vi "syncAIandAOat1MHz_v3.vi"() -> ()   [LabVIEW 2015]
uses:
  <vilib>/DAQmx/write.llb/DAQmx Write (Digital 1D Wfm NChan NSamp).vi
  <vilib>/DAQmx/write.llb/DAQmx Write (Analog 1D Wfm NChan NSamp).vi
  <vilib>/DAQmx/read.llb/DAQmx Read (Analog 2D I16 NChan NSamp).vi
  <vilib>/Waveform/DWDTOps.llb/DWDT Analog to Digital.vi
  <vilib>/DAQmx/create/channels.llb/DAQmx Create Channel (AO-Voltage-Basic).vi
  <vilib>/DAQmx/create/channels.llb/DAQmx Create Channel (AI-Voltage-Basic).vi
  <vilib>/DAQmx/create/channels.llb/DAQmx Create Channel (DO-Digital Output).vi
  <vilib>/DAQmx/configure/timing.llb/DAQmx Timing (Sample Clock).vi
  <vilib>/Waveform/DWDTOps.llb/DWDT Uncompress Digital.vi
  <vilib>/DAQmx/miscellaneous.llb/DAQmx Fill In Error Info.vi
  <vilib>/DAQmx/configure/trigger.llb/DAQmx Start Trigger (Digital Edge).vi
  <resource>/objmgr/daqmx.rc
panel:
  in  "numcyc":dbl=9.0 format="%#_13g"
  in  "finite":bool
  in  "cont":bool
  in  "error in 3":errorcluster caption="error in"
  in  "index (page)":i32
  out "XY Graph":T1(graph)
  in  "V":dbl=2.0 format="%#_13g"
  in  "AOrate":dbl=400000.0 format="%#_13g"
  in  "stop":bool
  out "Intensity Graph":sgl[][](graph)
  in  "error in 2":errorcluster caption="error in"
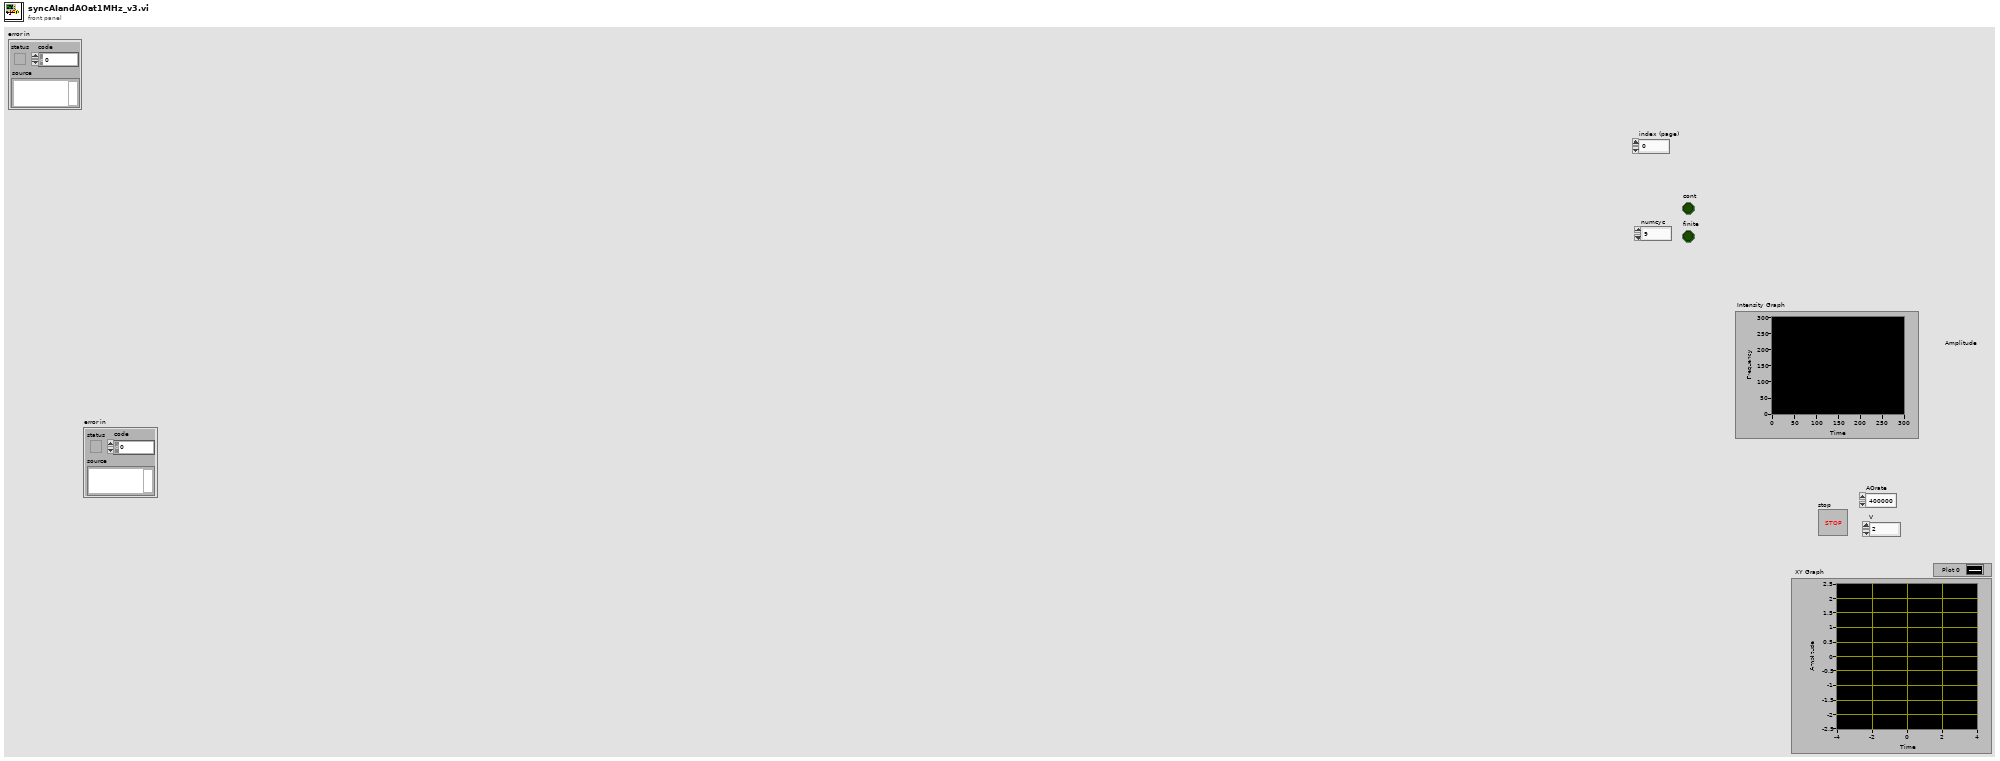
[diagram p1: front panel]
types:
  T1 = cluster{"X-WaveArray":dbl[], "Y-WaveArray":dbl[]}
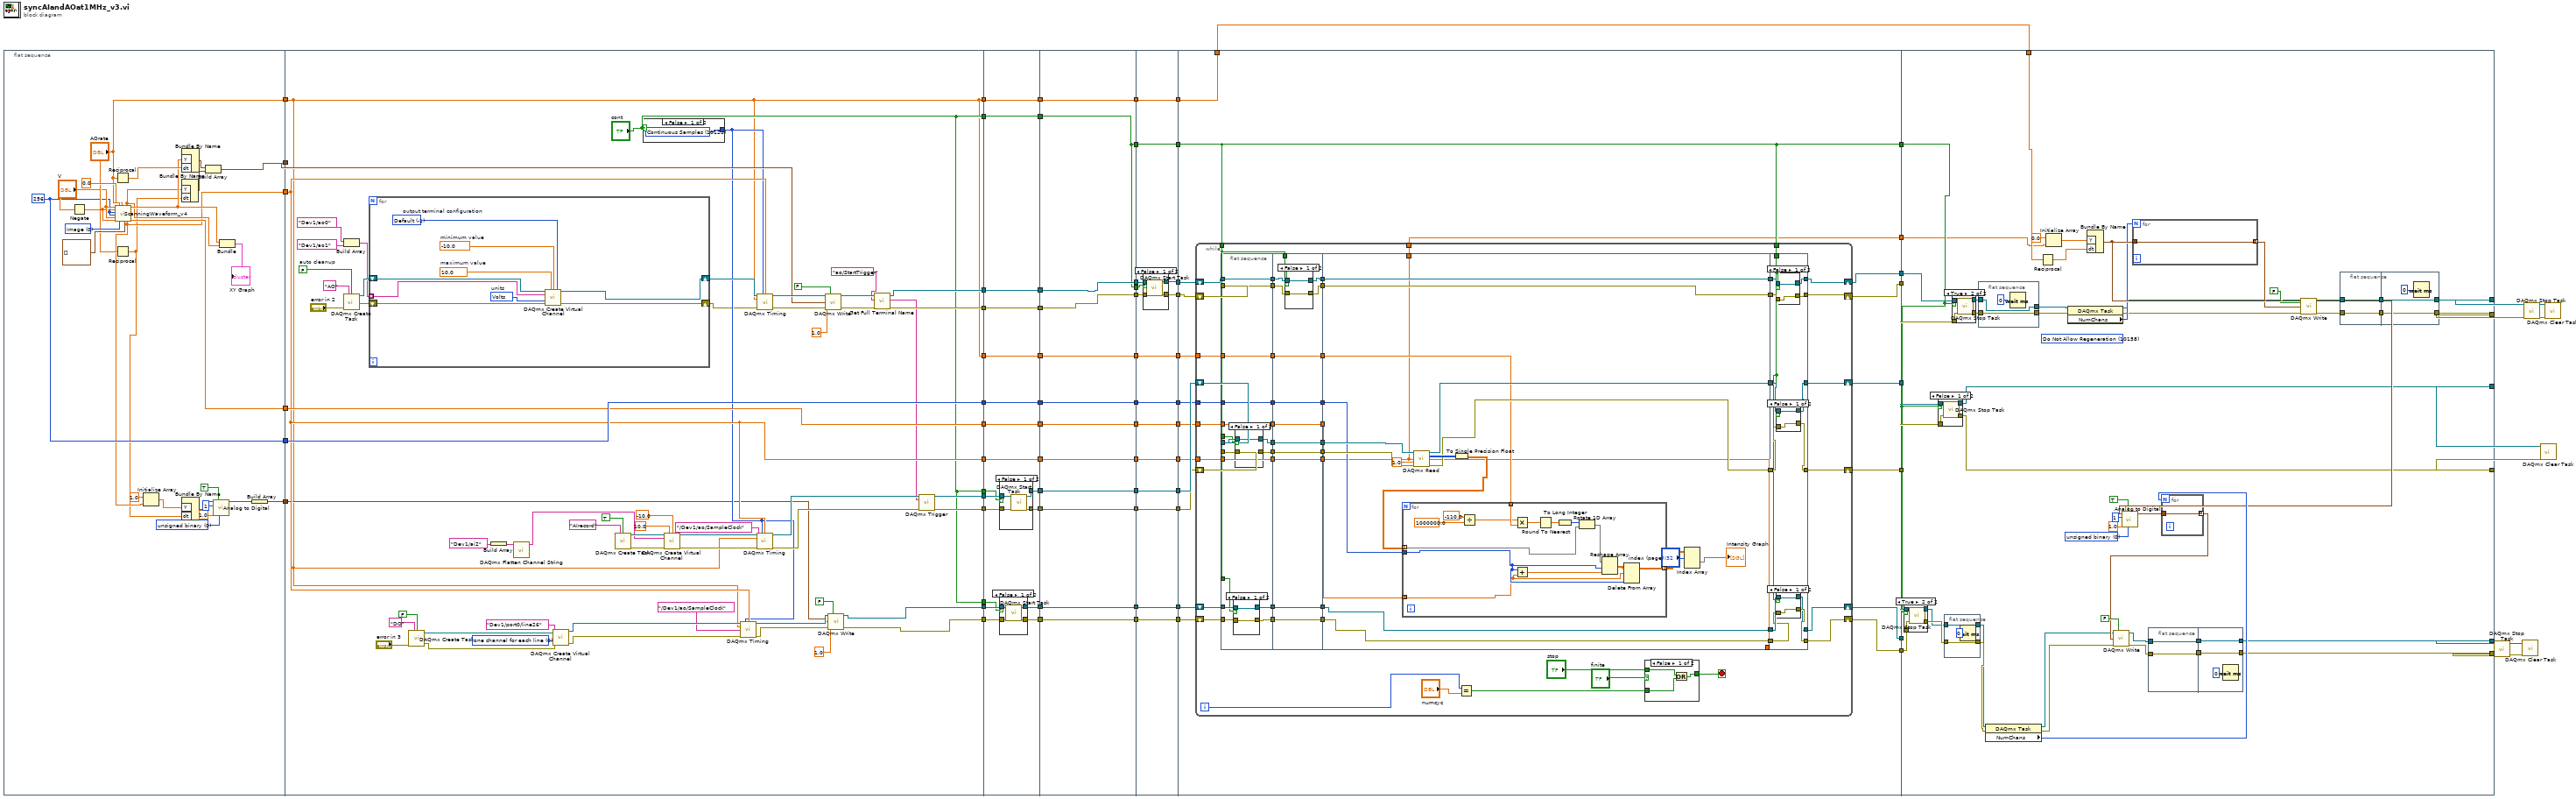
[diagram p0: block diagram]
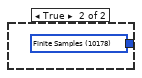
[diagram p2: hidden frame]
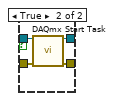
[diagram p7: hidden frame]
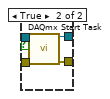
[diagram p8: hidden frame]
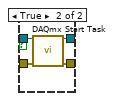
[diagram p9: hidden frame]
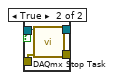
[diagram p10: hidden frame]
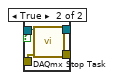
[diagram p11: hidden frame]
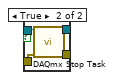
[diagram p12: hidden frame]
diagram:
  n1 = flat-sequence {
    tunnel: [w91] -> w76
    tunnel: [w87] -> w75
    tunnel: ["AOrate"] -> w74
    tunnel: [w93] -> w50
    tunnel: [w92] -> w45
    tunnel: [w77] -> w29
    tunnel: w76 -> [w150]
    tunnel: w75 -> [w118]
    tunnel: w74 -> [w103]
    tunnel: [w132] -> w73
    tunnel: [w138] -> w70
    tunnel: [w136] -> w69
    tunnel: [w118] -> w55
    tunnel: [w103] -> w51
    tunnel: w50 -> [w140]
    tunnel: [w140] -> w46
    tunnel: w45 -> [w139]
    tunnel: [w139] -> w41
    tunnel: [w131] -> w40
    tunnel: [w110] -> w37
    tunnel: [w109] -> w36
    tunnel: w29 -> [w108]
    tunnel: ["cont"] -> w14
    tunnel: ["cont"] -> w13
    tunnel: ["cont"] -> w12
    tunnel: [w103] -> w3
    tunnel: w73 -> [w191]
    tunnel: [w191] -> w72
    tunnel: [w190] -> w71
    tunnel: w70 -> [w189]
    tunnel: w69 -> [w188]
    tunnel: [w187] -> w63
    tunnel: [w186] -> w61
    tunnel: [w185] -> w56
    tunnel: w55 -> [w185]
    tunnel: [w184] -> w52
    tunnel: w51 -> [w184]
    tunnel: [w183] -> w47
    tunnel: w46 -> [w183]
    tunnel: [w182] -> w42
    tunnel: w41 -> [w182]
    tunnel: w40 -> [w190]
    tunnel: w37 -> [w181]
    tunnel: w36 -> [w180]
    tunnel: [w179] -> w33
    tunnel: [w178] -> w30
    tunnel: [w177] -> w15
    tunnel: w14 -> [w177]
    tunnel: w13 -> [w176]
    tunnel: w12 -> [w175]
    tunnel: [w174] -> w4
    tunnel: w3 -> [w174]
    tunnel: w72 -> [w209]
    tunnel: w71 -> [w208]
    tunnel: [w209] -> w68
    tunnel: [w208] -> w66
    tunnel: [w215] -> w64
    tunnel: w63 -> [w215]
    tunnel: [w214] -> w62
    tunnel: w61 -> [w214]
    tunnel: [w213] -> w57
    tunnel: w56 -> [w213]
    tunnel: [w212] -> w53
    tunnel: w52 -> [w212]
    tunnel: [w211] -> w48
    tunnel: w47 -> [w211]
    tunnel: [w210] -> w43
    tunnel: w42 -> [w210]
    tunnel: [w207] -> w34
    tunnel: w33 -> [w207]
    tunnel: [w206] -> w31
    tunnel: w30 -> [w206]
    tunnel: [w205] -> w16
    tunnel: w15 -> [w205]
    tunnel: [w205] -> w10
    tunnel: [w204] -> w5
    tunnel: w4 -> [w204]
    tunnel: w68 -> [w224]
    tunnel: [w222] -> w67
    tunnel: w66 -> [w223]
    tunnel: [w221] -> w65
    tunnel: w64 -> [w230]
    tunnel: w62 -> [w229]
    tunnel: [w230] -> w60
    tunnel: [w229] -> w59
    tunnel: [w228] -> w58
    tunnel: w57 -> [w228]
    tunnel: [w227] -> w54
    tunnel: w53 -> [w227]
    tunnel: [w226] -> w49
    tunnel: w48 -> [w226]
    tunnel: [w225] -> w44
    tunnel: w43 -> [w225]
    tunnel: [w220] -> w35
    tunnel: w34 -> [w220]
    tunnel: [w219] -> w32
    tunnel: w31 -> [w219]
    tunnel: w16 -> [w218]
    tunnel: [w217] -> w11
    tunnel: w10 -> [w217]
    tunnel: [w216] -> w6
    tunnel: w5 -> [w216]
    tunnel: w67 -> [w246]
    tunnel: w65 -> [w247]
    tunnel: w60 -> [w255]
    tunnel: w59 -> [w254]
    tunnel: w58 -> [w253]
    tunnel: w54 -> [w250]
    tunnel: w49 -> [w249]
    tunnel: w44 -> [w248]
    tunnel: w35 -> [w244]
    tunnel: w32 -> [w243]
    tunnel: [w252] -> w26
    tunnel: [w251] -> w25
    tunnel: [w239] -> w24
    tunnel: [w245] -> w23
    tunnel: [w242] -> w22
    tunnel: [w241] -> w21
    tunnel: w11 -> [w240]
    tunnel: [w240] -> w9
    tunnel: w6 -> [w238]
    tunnel: [w238] -> w2
    tunnel: [w237] -> w1
    tunnel: w26 -> [w431]
    tunnel: w25 -> [w429]
    tunnel: w24 -> [w441]
    tunnel: w23 -> [w440]
    tunnel: w22 -> [w435]
    tunnel: w21 -> [w434]
    tunnel: [w430] -> w8
    tunnel: [w428] -> w7
    tunnel: [w439] -> w20
    tunnel: [w438] -> w19
    tunnel: [w437] -> w17
    tunnel: [w436] -> w18
    tunnel: w9 -> [w427]
    tunnel: w2 -> [w426]
    tunnel: w1 -> [w421]
    frame #0 {
      w79 = u16 0 items=["unsigned binary", "offset binary", "2's complement"] ("data format (offset binary)")
      w93 = 256
      w101 = u16 0 items=["Image", "Fill Rectangle", "Fill Circle", "Draw Freeform", "Fill Freeform", "Ellipse Boundary", "Line"] ("Drawing Mode")
      n2 = Negate(x="V") -> (-x=w94:dbl)
      n3 = Reciprocal(x="AOrate") -> (1/x=w99:dbl)
      n4 = Reciprocal(x="AOrate") -> (1/x=w84:dbl)
      n5 = call "ScanningWaveform_v4.vi"("Vy-min"=w94, "Vy-max"="V", "yPixels/tPixels"=w93, "xPixels/rPixels"=w93, "Vx-min"=w94, "Vx-max"="V", "Drawing Mode"=w101, "Angle"=0.0, "AOrate"="AOrate", "Points"=cluster{"X":dbl, "Y":dbl}[] []) -> ("numPixels"=w87:dbl, "Y-WaveArray"=w89:dbl[], "P"=w92:dbl, "X-WaveArray"=w90:dbl[])  [unwired: 6 in]
      n6 = Initialize Array(1.0 ("element"), w87) -> (w85:dbl[])
      n7 = Bundle By Name("Y"=w89, "dt"=w84) -> (w97:waveform(dbl))  [unwired: 1 in]
      n8 = Bundle By Name("Y"=w90, "dt"=w99) -> (w98:waveform(dbl))  [unwired: 1 in]
      n9 = Bundle By Name("Y"=w85, "dt"=w84) -> (w83:waveform(dbl))  [unwired: 1 in]
      n10 = Build Array(w98, w97) -> (w91:waveform(dbl)[])
      n11 = call-poly <vilib>:"Analog to Digital.vi"("data format (offset binary)"=w79, "compress digital (T)"=TRUE, "full-scale range (pk-pk)"=1.0, "resolution (16 bit)"=1, "analog waveform"=w83) -> ("digital waveform"=w78:digitalwaveform)  [unwired: 3 in, 3 out]
      n12 = Bundle("X-WaveArray"=w90, "Y-WaveArray"=w89) -> (→"XY Graph":T1)  [unwired: 1 in]
      n13 = Build Array(w78) -> (w77:digitalwaveform[])
    }
    frame #1 {
      w121 = 0 items=["one channel for each line", "one channel for all lines"] ("line grouping")
      w160 = FALSE  # auto cleanup
      n14 = Build Array(tag "Dev1/ao0" ("physical channels"), tag "Dev1/ao1" ("physical channels")) -> (w151:tag[])
      n15 = call <vilib>:"DAQmx Create Task.vi"("new task name"="AO", "auto cleanup"=w160, "error in"="error in 2") -> ("task out"=w161:refnum<k21>, "error out"=w162:errorcluster)  [unwired: 11 in]
      n16 = for {
        shift-right: [w166] -> w157
        shift-left: w161 -> [w169]
        shift-right: [w165] -> w107
        shift-left: w162 -> [w168]
        tunnel: w151 -> [w167] mode=indexing
        w173 = -1 items=["Default"=-1, "RSE"=10083, "Differential"=10106, "Pseudodifferential"=12529]  # output terminal configuration
        w172 = 10348 items=["Volts"=10348, "From Custom Scale"=10065]  # units
        w171 = -10.0  # minimum value
        w170 = 10.0  # maximum value
        n17 = call-poly <vilib>:"DAQmx Create Virtual Channel.vi"("task in"=w169, "maximum value"=w170, "minimum value"=w171, "output terminal configuration"=w173, "physical channels"=w167, "units"=w172, "error in"=w168) -> ("task out"=w166:refnum<k21>, "error out"=w165:errorcluster)  [unwired: 7 in]
      }
      n18 = call <vilib>:"DAQmx Create Task.vi"("new task name"="DO", "auto cleanup"=FALSE, "error in"="error in 3") -> ("task out"=w125:refnum<k21>, "error out"=w120:errorcluster)  [unwired: 11 in]
      n19 = Build Array(tag "Dev1/ai2" ("physical channels")) -> (w129:tag[])
      n20 = call <vilib>:"DAQmx Flatten Channel String.vi"("names in"=w129) -> ("names out"=w127:string)  [unwired: 13 in, 1 out]
      n21 = call-poly <vilib>:"DAQmx Create Virtual Channel.vi"("task in"=w125, "lines"=tag "Dev1/port0/line26", "line grouping"=w121, "error in"=w120) -> ("task out"=w119:refnum<k21>, "error out"=w115:errorcluster)  [unwired: 10 in]
      n22 = call <vilib>:"DAQmx Create Task.vi"("new task name"="AIrecord", "auto cleanup"=TRUE) -> ("task out"=w143:refnum<k21>, "error out"=w144:errorcluster)  [unwired: 12 in]
      n23 = case shown="False" "cont" {
        tunnel: [w163 w164] -> w117
        frame False {
          w163 = 10123 items=["Finite Samples"=10178, "Continuous Samples"=10123, "Hardware Timed Single Point"=12522] ("sample mode")
        }
        frame True {
          w164 = 10178 items=["Finite Samples"=10178, "Continuous Samples"=10123, "Hardware Timed Single Point"=12522] ("sample mode")
        }
      }
      n24 = call-poly <vilib>:"DAQmx Create Virtual Channel.vi"("task in"=w143, "maximum value"=10.0, "minimum value"=-10.0, "physical channels"=w127, "error in"=w144) -> ("task out"=w149:refnum<k21>, "error out"=w148:errorcluster)  [unwired: 9 in]
      n25 = call-poly <vilib>:"DAQmx Timing.vi"("task/channels in"=w119, "sample mode"=w117, "samples per channel"=w118, "rate"=w103, "source"=tag "/Dev1/ao/SampleClock", "error in"=w115) -> ("task out"=w114:refnum<k21>, "error out"=w113:errorcluster)  [unwired: 8 in]
      n26 = call-poly <vilib>:"DAQmx Timing.vi"("task/channels in"=w149, "sample mode"=w117, "samples per channel"=w118, "rate"=w103, "source"=tag "/Dev1/ao/SampleClock", "error in"=w148) -> ("task out"=w141:refnum<k21>, "error out"=w137:errorcluster)  [unwired: 8 in]
      n27 = call-poly <vilib>:"DAQmx Timing.vi"("task/channels in"=w157, "sample mode"=w117, "samples per channel"=w118, "rate"=w103, "error in"=w107) -> ("task out"=w156:refnum<k21>, "error out"=w155:errorcluster)  [unwired: 2 in, 7 out]
      n28 = call-poly <vilib>:"DAQmx Write.vi"("task/channels in"=w156, "auto start"=FALSE, "data"=w150, "timeout"=1.0, "error in"=w155) -> ("task out"=w135:refnum<k21>, "error out"=w134:errorcluster)  [unwired: 8 in, 1 out]
      n29 = call-poly <vilib>:"DAQmx Write.vi"("task/channels in"=w114, "auto start"=FALSE, "data"=w108, "timeout"=1.0, "error in"=w113) -> ("task out"=w110:refnum<k21>, "error out"=w109:errorcluster)  [unwired: 8 in, 1 out]
      n30 = call "Get Full Terminal Name.vi"("error in"=w134, "Local Terminal Name"="ao/StartTrigger", "task/channels in"=w135) -> ("error out"=w131:errorcluster, "Terminal Name with Device Prefix"=w111:tag, "task out"=w132:refnum<k21>)  [unwired: 6 in]
      n31 = call-poly <vilib>:"DAQmx Trigger.vi"("task/channels in"=w141, "source"=w111, "error in"=w137) -> ("task out"=w138:refnum<k21>, "error out"=w136:errorcluster)  [unwired: 11 in]
    }
    frame #2 {
      n32 = case shown="False" w176 {
        tunnel: w189 -> [w201 w203]
        tunnel: w188 -> [w200 w202]
        tunnel: [w199 w203] -> w187
        tunnel: [w198 w202] -> w186
        frame False {
          n33 = call <vilib>:"DAQmx Start Task.vi"("task/channels in"=w201, "error in"=w200) -> ("task out"=w199:refnum<k21>, "error out"=w198:errorcluster)  [unwired: 12 in]
        }
        frame True {
        }
      }
      n34 = case shown="False" w175 {
        tunnel: w181 -> [w195 w197]
        tunnel: w180 -> [w194 w196]
        tunnel: [w193 w197] -> w179
        tunnel: [w192 w196] -> w178
        frame False {
          n35 = call <vilib>:"DAQmx Start Task.vi"("task/channels in"=w195, "error in"=w194) -> ("task out"=w193:refnum<k21>, "error out"=w192:errorcluster)  [unwired: 12 in]
        }
        frame True {
        }
      }
    }
    frame #3 {
    }
    frame #4 {
      n36 = case shown="False" w218 {
        tunnel: w224 -> [w234 w236]
        tunnel: w223 -> [w233 w235]
        tunnel: [w232 w236] -> w222
        tunnel: [w231 w235] -> w221
        frame False {
          n37 = call <vilib>:"DAQmx Start Task.vi"("task/channels in"=w234, "error in"=w233) -> ("task out"=w232:refnum<k21>, "error out"=w231:errorcluster)  [unwired: 12 in]
        }
        frame True {
        }
      }
    }
    frame #5 {
      n38 = while {
        tunnel: w253 -> [w304]
        tunnel: w250 -> [w301]
        tunnel: w249 -> [w300]
        tunnel: w248 -> [w299]
        shift-right: [w303] -> w252
        shift-left: w255 -> [w306]
        shift-right: [w302] -> w251
        shift-left: w254 -> [w305]
        tunnel: w240 -> [w260]
        tunnel: w240 -> [w259]
        shift-right: [w257] -> w239
        shift-left: w246 -> [w289]
        shift-right: [w288] -> w245
        shift-left: w247 -> [w287]
        shift-right: [w293] -> w242
        shift-left: w244 -> [w292]
        shift-right: [w291] -> w241
        shift-left: w243 -> [w290]
        tunnel: [w256] -> w237
        i -> [w297]
        stop <- w294 stop-if-true
        n39 = flat-sequence {
          tunnel: w287 -> [w321]
          tunnel: w289 -> [w322]
          tunnel: w290 -> [w319]
          tunnel: w292 -> [w320]
          tunnel: w299 -> [w323]
          tunnel: w300 -> [w324]
          tunnel: w301 -> [w325]
          tunnel: w304 -> [w326]
          tunnel: w305 -> [w315]
          tunnel: w306 -> [w316]
          tunnel: [w314] -> w277
          tunnel: [w326] -> w276
          tunnel: [w325] -> w275
          tunnel: [w324] -> w274
          tunnel: [w323] -> w273
          tunnel: [w318] -> w272
          tunnel: [w317] -> w271
          tunnel: [w322] -> w270
          tunnel: [w321] -> w269
          tunnel: [w313] -> w267
          tunnel: w260 -> [w312]
          tunnel: w260 -> [w311]
          tunnel: [w351] -> w286
          tunnel: [w350] -> w285
          tunnel: [w349] -> w284
          tunnel: [w348] -> w283
          tunnel: [w347] -> w282
          tunnel: [w346] -> w281
          tunnel: [w345] -> w280
          tunnel: [w344] -> w279
          tunnel: [w341] -> w278
          tunnel: w277 -> [w351]
          tunnel: w276 -> [w349]
          tunnel: w275 -> [w348]
          tunnel: w274 -> [w347]
          tunnel: w273 -> [w346]
          tunnel: w272 -> [w345]
          tunnel: w271 -> [w344]
          tunnel: w270 -> [w343]
          tunnel: w269 -> [w342]
          tunnel: [w340] -> w268
          tunnel: w267 -> [w350]
          tunnel: w260 -> [w339]
          tunnel: w286 -> [w374]
          tunnel: w285 -> [w373]
          tunnel: w284 -> [w358]
          tunnel: w283 -> [w368]
          tunnel: w282 -> [w367]
          tunnel: w281 -> [w366]
          tunnel: w280 -> [w362]
          tunnel: w279 -> [w361]
          tunnel: w278 -> [w360]
          tunnel: w268 -> [w359]
          tunnel: [w371] -> w266
          tunnel: [w370] -> w265
          tunnel: [w362] -> w264
          tunnel: [w361] -> w263
          tunnel: [w360] -> w262
          tunnel: [w359] -> w261
          tunnel: [w358] -> _
          tunnel: [w358] -> w256
          tunnel: [w399] -> w288
          tunnel: [w400] -> w257
          tunnel: [w392] -> w291
          tunnel: [w391] -> w293
          tunnel: [w395] -> w302
          tunnel: [w397] -> w303
          tunnel: w266 -> [w398]
          tunnel: w265 -> [w396]
          tunnel: w264 -> [w394]
          tunnel: w263 -> [w393]
          tunnel: w262 -> [w402]
          tunnel: w261 -> [w401]
          tunnel: w259 -> [w390]
          frame #0 {
            n40 = case shown="False" w311 {
              tunnel: w320 -> [w334 w338]
              tunnel: w319 -> [w333 w337]
              tunnel: [w334 w336] -> w318
              tunnel: [w333 w335] -> w317
              frame False {
              }
              frame True {
                n41 = call <vilib>:"DAQmx Start Task.vi"("task/channels in"=w338, "error in"=w337) -> ("task out"=w336:refnum<k21>, "error out"=w335:errorcluster)  [unwired: 12 in]
              }
            }
            n42 = case shown="False" w312 {
              tunnel: w316 -> [w328 w332]
              tunnel: w315 -> [w327 w331]
              tunnel: [w328 w330] -> w314
              tunnel: [w327 w329] -> w313
              frame False {
              }
              frame True {
                n43 = call <vilib>:"DAQmx Start Task.vi"("task/channels in"=w332, "error in"=w331) -> ("task out"=w330:refnum<k21>, "error out"=w329:errorcluster)  [unwired: 12 in]
              }
            }
          }
          frame #1 {
            n44 = case shown="False" w339 {
              tunnel: w343 -> [w353 w357]
              tunnel: w342 -> [w352 w356]
              tunnel: [w353 w355] -> w341
              tunnel: [w352 w354] -> w340
              frame False {
              }
              frame True {
                n45 = call <vilib>:"DAQmx Start Task.vi"("task/channels in"=w357, "error in"=w356) -> ("task out"=w355:refnum<k21>, "error out"=w354:errorcluster)  [unwired: 12 in]
              }
            }
          }
          frame #2 {
            n46 = call-poly <vilib>:"DAQmx Read.vi"("task/channels in"=w374, "number of samples per channel"=w358, "timeout"=1.0, "error in"=w373) -> ("task out"=w371:refnum<k21>, "data"=w375:i16[][], "error out"=w370:errorcluster)  [unwired: 9 in]
            n47 = To Single Precision Float(number=w375) -> (single precision float=w369:sgl[][])
            n48 = for {
              tunnel: w369 -> [w389] mode=indexing
              tunnel: w368 -> [w388]
              tunnel: w367 -> [w387]
              tunnel: w366 -> [w386]
              tunnel: [w376] -> w365 mode=indexing
              n49 = Divide(x=-110.0, y=1000000.0) -> (x/y=w382:dbl)
              n50 = Multiply(x=w382, y=w388) -> (x*y=w378:dbl)
              n51 = Add(x=w387, y=w386) -> (x+y=w377:dbl)
              n52 = Round To Nearest(number=w378) -> (nearest integer value=w381:dbl)
              n53 = To Long Integer(number=w381) -> (32bit integer=w379:i32)
              n54 = Rotate 1D Array(1:w389, 2:w379) -> (0:w380:sgl[])
              n55 = Reshape Array(w380, w387, w377) -> (w385:sgl[][])
              n56 = Delete From Array(array=w385, length=w386, index (col)=w387) -> (array with subset deleted=w376:sgl[][])  [unwired: 1 in, 1 out]
            }
            n57 = Index Array(array=w365, index (dim 0)="index (page)") -> (element=→"Intensity Graph":sgl[][])  [unwired: 2 in]
          }
          frame #3 {
            n58 = case shown="False" w390 {
              tunnel: [w415 w420] -> w399
              tunnel: [w416 w419] -> w400
              tunnel: w402 -> [w416 w418]
              tunnel: w401 -> [w415 w417]
              frame False {
              }
              frame True {
                n59 = call <vilib>:"DAQmx Stop Task.vi"("task/channels in"=w418, "error in"=w417) -> ("task out"=w419:refnum<k21>, "error out"=w420:errorcluster)  [unwired: 12 in]
              }
            }
            n60 = case shown="False" w390 {
              tunnel: [w409 w414] -> w395
              tunnel: [w410 w413] -> w397
              tunnel: w398 -> [w410 w412]
              tunnel: w396 -> [w409 w411]
              frame False {
              }
              frame True {
                n61 = call <vilib>:"DAQmx Stop Task.vi"("task/channels in"=w412, "error in"=w411) -> ("task out"=w413:refnum<k21>, "error out"=w414:errorcluster)  [unwired: 12 in]
              }
            }
            n62 = case shown="False" w390 {
              tunnel: [w403 w408] -> w392
              tunnel: [w404 w407] -> w391
              tunnel: w394 -> [w404 w406]
              tunnel: w393 -> [w403 w405]
              frame False {
              }
              frame True {
                n63 = call <vilib>:"DAQmx Stop Task.vi"("task/channels in"=w406, "error in"=w405) -> ("task out"=w407:refnum<k21>, "error out"=w408:errorcluster)  [unwired: 12 in]
              }
            }
          }
        }
        n64 = Equal?(x=w297, y="numcyc") -> (x = y?=w295:bool)
        n65 = case shown="False" "finite" {
          tunnel: "stop" -> [w309 w310]
          tunnel: w295 -> [w308 _]
          tunnel: [w307 w310] -> w294
          frame False {
            n66 = Or(x=w309, y=w308) -> (x .or. y?=w307:bool)
          }
          frame True {
          }
        }
      }
    }
    frame #6 {
      w453 = u16 0 items=["unsigned binary", "offset binary", "2's complement"] ("data format (offset binary)")
      (unwired) 10158 items=["Allow Regeneration"=10097, "Do Not Allow Regeneration"=10158] ("RegenMode")
      n67 = case shown="True" w427 {
        tunnel: [w477 w482] -> w433
        tunnel: [w478 w481] -> w432
        tunnel: w435 -> [w478 w480]
        tunnel: w434 -> [w477 w479]
        frame False {
        }
        frame True {
          n68 = call <vilib>:"DAQmx Stop Task.vi"("task/channels in"=w480, "error in"=w479) -> ("task out"=w481:refnum<k21>, "error out"=w482:errorcluster)  [unwired: 12 in]
        }
      }
      n69 = case shown="False" w427 {
        tunnel: [w474 w475] -> w428
        tunnel: [w473 w476] -> w430
        tunnel: w431 -> [w472 w476]
        tunnel: w429 -> [w471 w475]
        frame False {
          n70 = call <vilib>:"DAQmx Stop Task.vi"("task/channels in"=w472, "error in"=w471) -> ("task out"=w473:refnum<k21>, "error out"=w474:errorcluster)  [unwired: 12 in]
        }
        frame True {
        }
      }
      n71 = flat-sequence {
        tunnel: [w491] -> w459
        tunnel: w433 -> [w493]
        tunnel: [w493] -> w460
        tunnel: w432 -> [w491]
        frame #0 {
          n72 = Wait (ms)(milliseconds to wait=u32 0) -> ()  [unwired: 1 out]
        }
      }
      n73 = case shown="True" w427 {
        tunnel: [w483 w488] -> w445
        tunnel: [w484 w487] -> w444
        tunnel: w441 -> [w484 w486]
        tunnel: w440 -> [w483 w485]
        frame False {
        }
        frame True {
          n74 = call <vilib>:"DAQmx Stop Task.vi"("task/channels in"=w486, "error in"=w485) -> ("task out"=w487:refnum<k21>, "error out"=w488:errorcluster)  [unwired: 12 in]
        }
      }
      n75 = flat-sequence {
        tunnel: w444 -> [w501]
        tunnel: [w501] -> w446
        tunnel: w445 -> [w500]
        tunnel: [w500] -> w456
        frame #0 {
          n76 = Wait (ms)(milliseconds to wait=u32 0) -> ()  [unwired: 1 out]
        }
      }
      n77 = property class="DAQmx Task"(reference=w459, error in=w460) -> (reference out=w423:refnum<k21>, error out=w422:errorcluster, "NumChans"=w464:u32)
      n78 = Reciprocal(x=w426) -> (1/x=w461:dbl)
      n79 = Initialize Array(0.0 ("element"), w421) -> (w454:dbl[])
      n80 = property class="DAQmx Task"(reference=w446, error in=w456) -> (reference out=w425:refnum<k21>, error out=w424:errorcluster, "NumChans"=w458:u32)
      n81 = Bundle By Name("Y"=w454, "dt"=w461) -> (w462:waveform(dbl))  [unwired: 1 in]
      n82 = call-poly <vilib>:"Analog to Digital.vi"("data format (offset binary)"=w453, "compress digital (T)"=TRUE, "full-scale range (pk-pk)"=1.0, "resolution (16 bit)"=1, "analog waveform"=w462) -> ("digital waveform"=w463:digitalwaveform)  [unwired: 3 in, 3 out]
      n83 = for {
        N: w458 -> [_]
        tunnel: w462 -> [w490]
        tunnel: [w490] -> w457 mode=indexing
      }
      n84 = flat-sequence {
        tunnel: [w495] -> w468
        tunnel: [w494] -> w467
        tunnel: w448 -> [w495]
        tunnel: w447 -> [w494]
        tunnel: [w497] -> w437
        tunnel: [w498] -> w436
        tunnel: w468 -> [w498]
        tunnel: w467 -> [w497]
        frame #0 {
        }
        frame #1 {
          n85 = Wait (ms)(milliseconds to wait=u32 0) -> ()  [unwired: 1 out]
        }
      }
      n86 = for {
        N: w464 -> [_]
        tunnel: w463 -> [w489]
        tunnel: [w489] -> w465 mode=indexing
      }
      n87 = call-poly <vilib>:"DAQmx Write.vi"("task/channels in"=w423, "auto start"=FALSE, "data"=w465, "error in"=w422) -> ("task out"=w448:refnum<k21>, "error out"=w447:errorcluster)  [unwired: 9 in, 1 out]
      n88 = call-poly <vilib>:"DAQmx Write.vi"("task/channels in"=w425, "auto start"=FALSE, "data"=w457, "error in"=w424) -> ("task out"=w442:refnum<k21>, "error out"=w443:errorcluster)  [unwired: 9 in, 1 out]
      n89 = flat-sequence {
        tunnel: [w503] -> w470
        tunnel: [w502] -> w469
        tunnel: w442 -> [w503]
        tunnel: w443 -> [w502]
        tunnel: [w505] -> w438
        tunnel: [w506] -> w439
        tunnel: w470 -> [w506]
        tunnel: w469 -> [w505]
        frame #0 {
        }
        frame #1 {
          n90 = Wait (ms)(milliseconds to wait=u32 0) -> ()  [unwired: 1 out]
        }
      }
    }
  }
  n91 = call <vilib>:"DAQmx Stop Task.vi"("task/channels in"=w18, "error in"=w17) -> ("task out"=w27:refnum<k21>, "error out"=w28:errorcluster)  [unwired: 12 in]
  n92 = call <vilib>:"DAQmx Clear Task.vi"("task in"=w27, "error in"=w28) -> ()  [unwired: 13 in, 1 out]
  n93 = call <vilib>:"DAQmx Stop Task.vi"("task/channels in"=w20, "error in"=w19) -> ("task out"=w39:refnum<k21>, "error out"=w38:errorcluster)  [unwired: 12 in]
  n94 = call <vilib>:"DAQmx Clear Task.vi"("task in"=w8, "error in"=w7) -> ()  [unwired: 13 in, 1 out]
  n95 = call <vilib>:"DAQmx Clear Task.vi"("task in"=w39, "error in"=w38) -> ()  [unwired: 13 in, 1 out]
